vi "加标回收启动 (子VI).vi"(11 "启动参数":T1(ring)=enum."CODCr") -> (0 "error out":T2={"status"=FALSE, "代码"=4, "source"=""} caption="错误输出" {"代码" items=["执行成功"=1, "执行失败，但不知道原因"=2, "命令请求条件错误"=3, "通讯超时"=4, "系统繁忙不能执行"=5, "系统故障"=6, "没有数据"=100]})   [LabVIEW 2016]
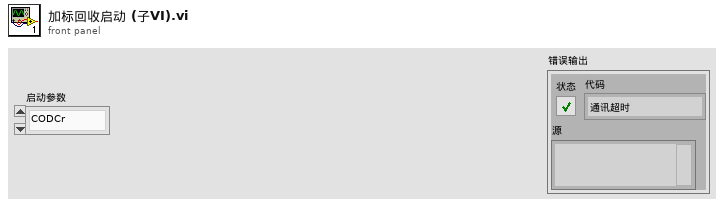
[diagram p1: front panel]
types:
  T1 = enum16{"未选择", "CODMn", "氨氮", "总磷", "总氮", "CODCr"}
  T2 = cluster{"status":bool, "代码":u16, "source":string}
  T3 = typedef "质控单元V4.lvlib/测试子流程.ctl" = enum16{"水样测试（润洗采样分开）", "水样测试（润洗采样合并）", "水样测试（不启动采配水）", "加标回收（润洗采样分开）", "加标回收（润洗采样合并）", "加标回收（不启动采配水）", "集成干预测试", "平行样测试", "平行样测试（不启动采配水）"}
  T4 = typedef "质控单元V4.lvlib/质控slave id.ctl" = enum16{"null", "氨氮", "总磷", "总氮", "CODMn", "CODCr"}
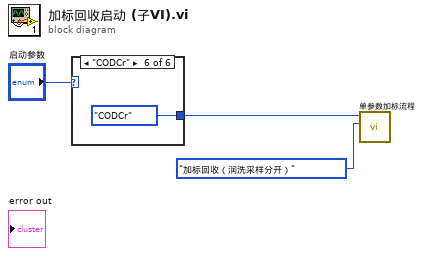
[diagram p0: block diagram]
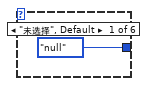
[diagram p2: hidden frame]
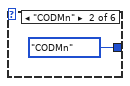
[diagram p3: hidden frame]
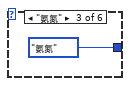
[diagram p4: hidden frame]
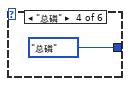
[diagram p5: hidden frame]
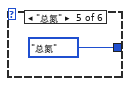
[diagram p6: hidden frame]
diagram:
  n1 = case shown="\"CODCr\"" "启动参数" {
    tunnel: [质控slave_id."null" ("Slave ID") 质控slave_id."CODMn" ("Slave ID") 质控slave_id."氨氮" ("Slave ID") 质控slave_id."总磷" ("Slave ID") 质控slave_id."总氮" ("Slave ID") 质控slave_id."CODCr" ("Slave ID")] -> w2
    frame "未选择", Default {
    }
    frame "CODMn" {
    }
    frame "氨氮" {
    }
    frame "总磷" {
    }
    frame "总氮" {
    }
    frame "CODCr" {
    }
  }
  n2 = call "单参数加标流程.vi"("流程类型"=测试子流程."加标回收（润洗采样分开）", "Slave ID"=w2) -> ()  [unwired: 10 in]
